vi "20210709_Scan with scanning mirror_draw graph_subVI.vi"(0 "X center (V)":dbl min=-200.0 max=300.0, 1 "Y center (V)":dbl min=-200.0 max=300.0, 2 "Bool Refnum":refnum<vi>, 4 "X Scan range (V)":dbl=0.2 min=-200.0 max=300.0, 5 "Y Scan range (V)":dbl=0.2 min=-200.0 max=300.0, 6 "X data number(Ao1)":i32=150, 7 "Y data number(Ao0)":i32=150, 8 "DigNum Refnum 7":refnum<vi>, 9 "DigNum Refnum 4":refnum<vi>, 10 "DigNum Refnum 3":refnum<vi>, 11 "DigNum Refnum 8":refnum<vi>, 12 "DigNum Refnum 5":refnum<vi>, 13 "DigNum Refnum 6":refnum<vi>, 14 "IntGraph Refnum":refnum<vi>, 18 "DigNum Refnum":refnum<vi>, 19 "DigNum Refnum 2":refnum<vi>) -> (15 "Intensity Graph":dbl[][](graph))   [LabVIEW 2015]
uses:
  Libraries/SR400/Public/Typedefs/Counter.ctl
  <vilib>/Analysis/1siggen.llb/Ramp Pattern by Samples.vi
  <vilib>/Analysis/NI_AALBase.lvlib
  Libraries/SR400/SR400.lvlib
panel:
  in  "file path":path
  out "STOP SCAN":bool
  in  "Count Time Set":dbl[unit]=0.01
  in  "# of average":i32=1
  in  "Dwell time (ms)":i32=2
  in  "Time delay bet. movement\n& measurement (ms)":i32=1
  out "Max Value":dbl format="%#.2p"
  out "Max Y (V)":dbl format="%#.5f"
  out "Max X (V)":dbl format="%#.5f"
  out "Counts":dbl
  out "ao1_V":dbl
  out "ao1_index":i32
  out "ao0_V":dbl
  out "ao0_index":i32
  in  "VISA resource name":refnum<visa-resource-name>="GPIB0::18::INSTR"
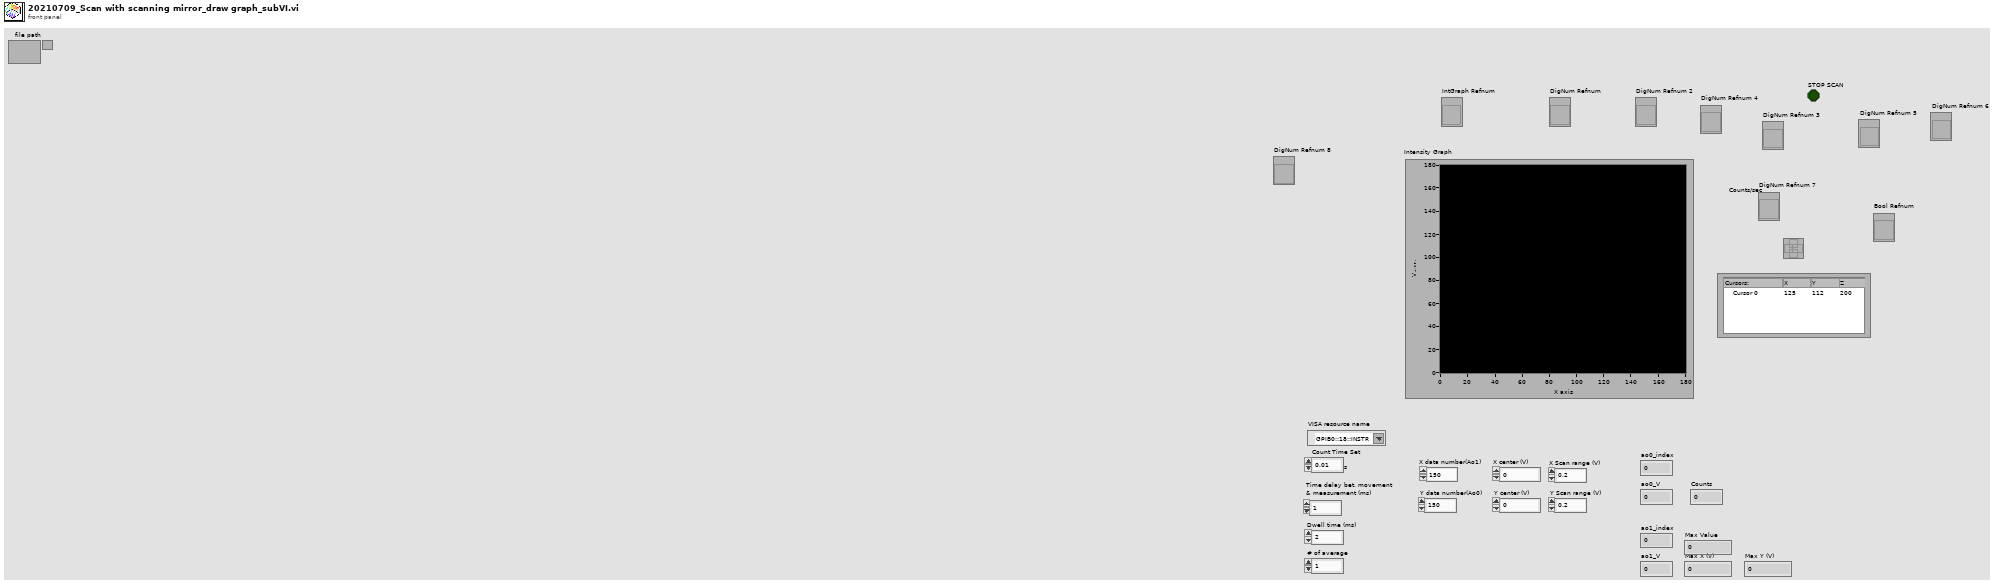
[diagram p1: front panel]
types:
  T1 = enum16{"open", "open or create", "create or replace", "create", "open (read only)"}
  T2 = typedef "SR400.lvlib/Counter.ctl" = enum16{"Counter A", "Counter B", "Counter T"}
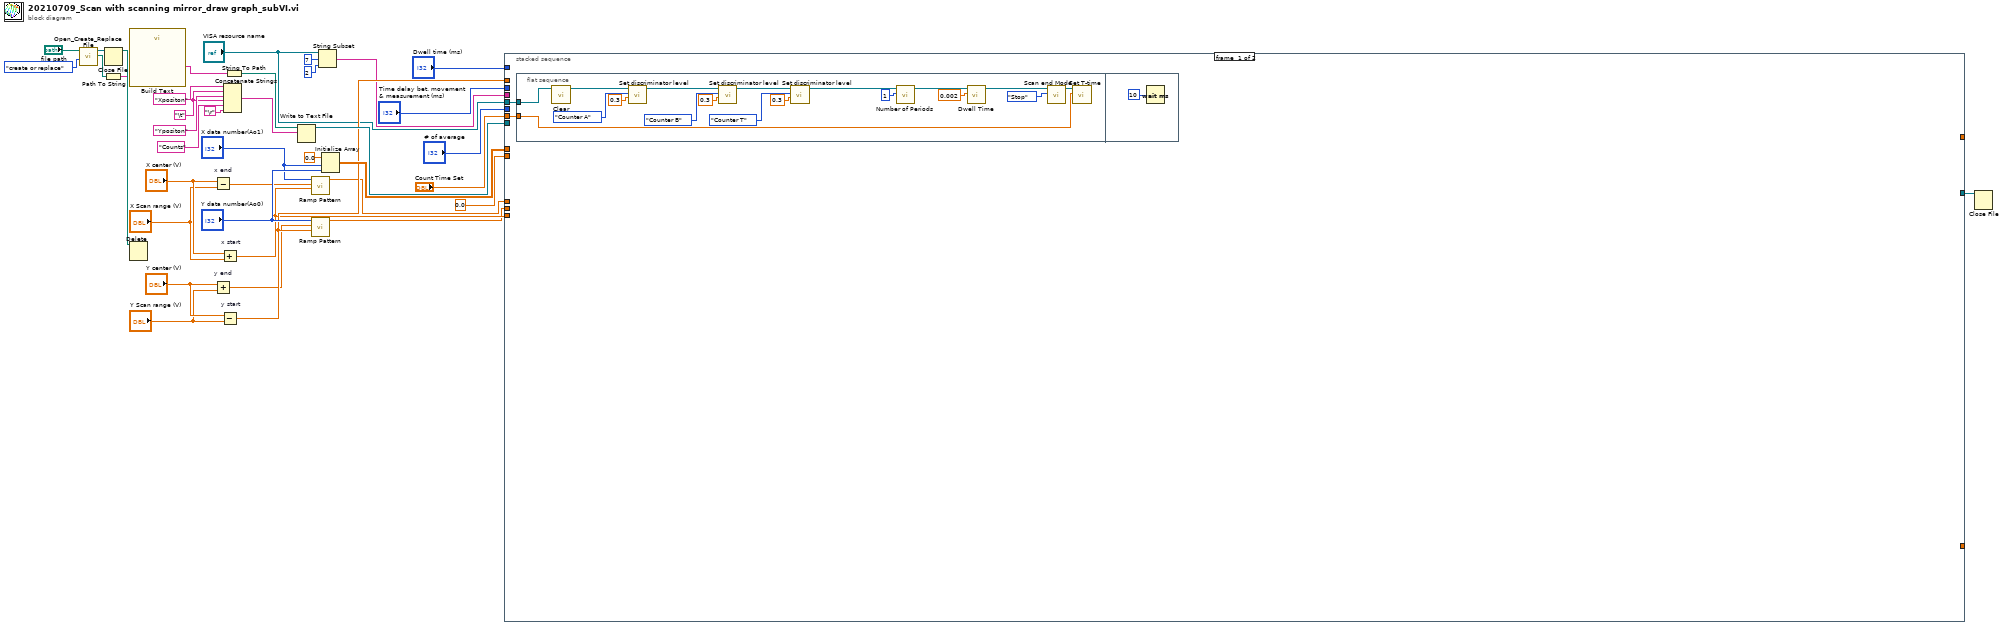
[diagram p0: block diagram]
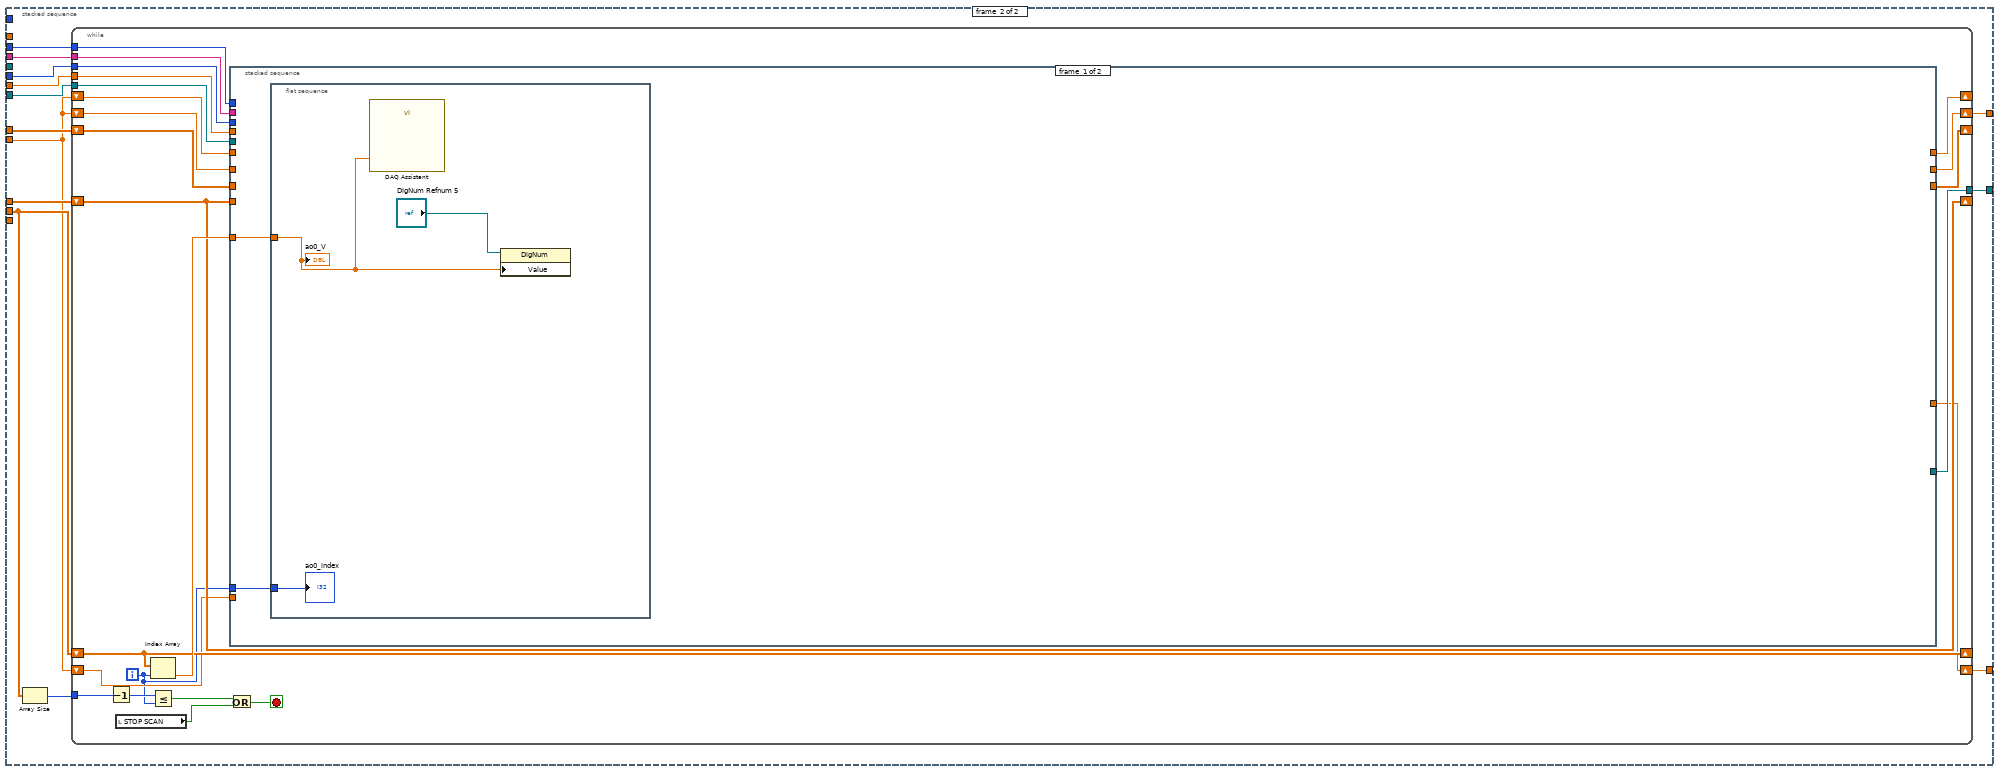
[diagram p2: hidden frame]
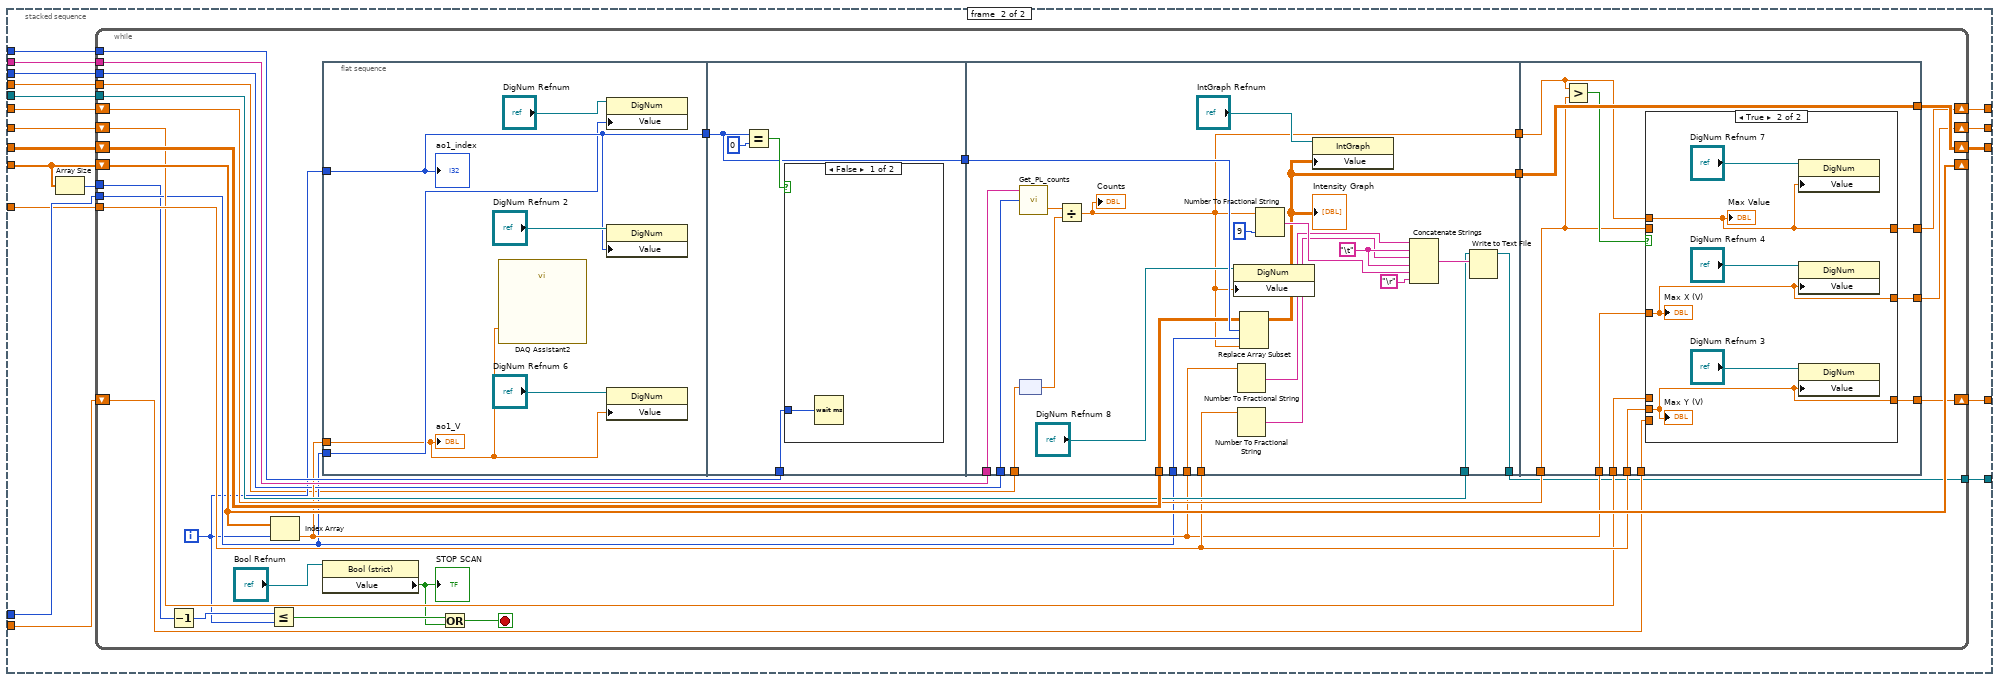
[diagram p3: hidden frame]
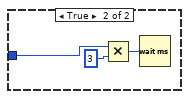
[diagram p4: hidden frame]
diagram:
  w31 = "\t"
  n1 = call <vilib>:"Open_Create_Replace File.vi"("function (open:0)"=T1."create or replace", "file path"="file path") -> ("new file path"=w4:path, "refnum"=w6:refnum<file>)  [unwired: 6 in, 2 out]
  n2 = Path To String(path=w4) -> (string=w3:string)
  n3 = Close File(refnum=w6) -> (path=w5:path)  [unwired: 1 in, 1 out]
  n4 = call "Build Text"("a"=w3) -> ("Result"=w2:string)  [unwired: 13 in, 1 out]
  n5 = Delete(path (use dialog)=w5) -> ()  [unwired: 4 in, 3 out]
  n6 = Subtract "x end"(x="X center (V)", y="X Scan range (V)") -> (x-y=w21:dbl)
  n7 = Add "y end"(x="Y center (V)", y="Y Scan range (V)") -> (x+y=w22:dbl)
  n8 = Add "x start"(x="X center (V)", y="X Scan range (V)") -> (x+y=w20:dbl)
  n9 = Subtract "y start"(x="Y center (V)", y="Y Scan range (V)") -> (x-y=w23:dbl)
  n10 = Concatenate Strings("Xpositon" ("string"), w31, "Ypositon" ("string"), w31, "Counts" ("string"), "\r") -> (w34:string)
  n11 = String To Path(string=w2) -> (path=w1:path)
  n12 = Write to Text File(file (use dialog)=w1, text=w34) -> (refnum out=w28:refnum<file>)  [unwired: 2 in, 2 out]
  n13 = call-poly <vilib>:"Ramp Pattern.vi"("start"=w20, "end"=w21, "samples"="X data number(Ao1)") -> ("Ramp Pattern"=w14:dbl[])  [unwired: 7 in, 1 out]
  n14 = call-poly <vilib>:"Ramp Pattern.vi"("start"=w23, "end"=w22, "samples"="Y data number(Ao0)") -> ("Ramp Pattern"=w13:dbl[])  [unwired: 7 in, 1 out]
  n15 = String Subset(string="VISA resource name", offset (0)=7, length (rest)=2 ("length (rest)")) -> (substring=w10:string)
  n16 = Initialize Array(0.0, "X data number(Ao1)", "Y data number(Ao0)") -> (w35:dbl[][])
  n17 = stacked-sequence {
    tunnel: w13 -> [_ w73]
    tunnel: w14 -> [_ w72]
    tunnel: "Time delay bet. movement\n& measurement (ms)" -> [_ w71]
    tunnel: w10 -> [_ w70]
    tunnel: w35 -> [_ w69]
    tunnel: w28 -> [_ w68]
    tunnel: [_ w67] -> w27
    tunnel: w20 -> [_ _]
    tunnel: w23 -> [_ _]
    tunnel: 0.0 -> [_ w66]
    tunnel: "Dwell time (ms)" -> [_ _]
    tunnel: [_ w65] -> _
    tunnel: [_ w64] -> _
    tunnel: "# of average" -> [_ w63]
    tunnel: "Count Time Set" -> [w41 w61]
    tunnel: "VISA resource name" -> [w40 _]
    frame #0 {
      n18 = flat-sequence {
        tunnel: w41 -> [w43]
        tunnel: w40 -> [w42]
        frame #0 {
          n19 = call "Clear.vi"("VISA resource name"=w42) -> ("VISA resource name out"=w59:refnum<visa-resource-name>)  [unwired: 9 in, 1 out]
          n20 = call "Set discriminator level.vi"("Level (-0.034 V)"=0.3, "Discriminator (def: A)"=Counter."Counter A", "VISA resource name"=w59) -> ("VISA resource name out"=w56:refnum<visa-resource-name>)  [unwired: 7 in, 1 out]
          n21 = call "Set discriminator level.vi"("Level (-0.034 V)"=0.3, "Discriminator (def: A)"=Counter."Counter B", "VISA resource name"=w56) -> ("VISA resource name out"=w53:refnum<visa-resource-name>)  [unwired: 7 in, 1 out]
          n22 = call "Set discriminator level.vi"("Level (-0.034 V)"=0.3, "Discriminator (def: A)"=Counter."Counter T", "VISA resource name"=w53) -> ("VISA resource name out"=w50:refnum<visa-resource-name>)  [unwired: 7 in, 1 out]
          n23 = call "Number of Periods.vi"("# of periods (def: 1)"=1, "VISA resource name"=w50) -> ("VISA resource name out"=w48:refnum<visa-resource-name>)  [unwired: 8 in, 1 out]
          n24 = call "Dwell Time.vi"("Dwell time (0.002 s)"=0.002, "VISA resource name"=w48) -> ("VISA resource name out"=w46:refnum<visa-resource-name>)  [unwired: 8 in, 1 out]
          n25 = call "Scan end Mode.vi"("Scan End Mode (Def: Stop)"=enum16{"Stop", "Start"}."Stop", "VISA resource name"=w46) -> ("VISA resource name out"=w44:refnum<visa-resource-name>)  [unwired: 8 in, 1 out]
          n26 = call "Set T-time.vi"("Count Time Set"=w43, "VISA resource name"=w44) -> ()  [unwired: 5 in, 3 out]
        }
        frame #1 {
          n27 = Wait (ms)(milliseconds to wait=u32 10) -> ()  [unwired: 1 out]
        }
      }
    }
    frame #1 {
      n28 = Array Size(array=w73) -> (size(s)=w62:i32)
      n29 = while {
        shift-right: [w95] -> _
        shift-left: w73 -> [w95]
        shift-right: [w94] -> _
        shift-left: w72 -> [w94]
        tunnel: w71 -> [w93]
        tunnel: w70 -> [w92]
        shift-right: [w89] -> _
        shift-left: w69 -> [w91]
        tunnel: w68 -> [w90]
        tunnel: [w88] -> w67
        shift-right: [w87] -> w64
        shift-left: w66 -> [w82]
        shift-right: [w85] -> _
        shift-left: w66 -> [w83]
        shift-right: [w86] -> w65
        shift-left: w66 -> [w84]
        tunnel: w63 -> [w81]
        tunnel: w62 -> [w80]
        tunnel: w61 -> [w74]
        i -> [w78]
        stop <- w75 stop-if-true
        n30 = Decrement(x=w80) -> (x-1=w79:i32)
        n31 = local read "STOP SCAN"() -> (w76:bool)
        n32 = Index Array(array=w95, index=w78) -> (element=w96:dbl)
        n33 = Less Or Equal?(x=w79, y=w78) -> (x <= y?=w77:bool)
        n34 = stacked-sequence {
          tunnel: w96 -> [w98 w114]
          tunnel: w94 -> [_ w119]
          tunnel: w93 -> [_ w118]
          tunnel: w78 -> [w97 w116]
          tunnel: w92 -> [_ w117]
          tunnel: w91 -> [_ w115]
          tunnel: w90 -> [_ w113]
          tunnel: [_ w112] -> w89
          tunnel: [_ w111] -> w88
          tunnel: [_ w110] -> w87
          tunnel: [_ w109] -> w86
          tunnel: [_ w108] -> w85
          tunnel: w84 -> [_ w107]
          tunnel: w83 -> [_ w106]
          tunnel: w82 -> [_ w105]
          tunnel: w81 -> [_ w104]
          tunnel: w74 -> [_ w102]
          frame #0 {
            n35 = flat-sequence {
              tunnel: w98 -> [w99]
              tunnel: w97 -> [w101]
              frame #0 {
                n36 = call "DAQ Assistant"("data"=w99) -> ()  [unwired: 17 in, 2 out]
                n37 = property class="DigNum"(reference="DigNum Refnum 5", "Value"=w99) -> ()  [unwired: 1 in, 2 out]
                "ao0_V" <- w99
                "ao0_index" <- w101
              }
            }
          }
          frame #1 {
            n38 = Array Size(array=w119) -> (size(s)=w103:i32)
            n39 = while {
              shift-right: [w148] -> _
              shift-left: w119 -> [w148]
              tunnel: w118 -> [w147]
              tunnel: w117 -> [w146]
              tunnel: w116 -> [w128]
              shift-right: [w143] -> w112
              shift-left: w115 -> [w144]
              tunnel: w114 -> [w137]
              tunnel: w113 -> [w142]
              shift-right: [w139] -> w108
              shift-left: w106 -> [w138]
              shift-right: [w135] -> w110
              shift-left: w105 -> [w133]
              shift-right: [w134] -> w109
              shift-left: w107 -> [w132]
              tunnel: [w131] -> w111
              tunnel: w104 -> [w129]
              tunnel: w103 -> [w127]
              tunnel: w102 -> [w120]
              i -> [w125]
              stop <- w123 stop-if-true
              n40 = Decrement(x=w127) -> (x-1=w126:i32)
              n41 = Less Or Equal?(x=w126, y=w125) -> (x <= y?=w124:bool)
              n42 = Index Array(array=w148, index=w125) -> (element=w136:dbl)
              n43 = flat-sequence {
                tunnel: w136 -> [w149]
                tunnel: w125 -> [w152]
                tunnel: [w152] -> w130
                tunnel: w128 -> [w151]
                tunnel: w147 -> [w155]
                tunnel: [w157] -> w145
                tunnel: w130 -> [w157]
                tunnel: w146 -> [w171]
                tunnel: w145 -> [w185]
                tunnel: w128 -> [w184]
                tunnel: w144 -> [w183]
                tunnel: w136 -> [w176]
                tunnel: w137 -> [w175]
                tunnel: w142 -> [w173]
                tunnel: [w168] -> w141
                tunnel: [w164] -> w140
                tunnel: [w172] -> w131
                tunnel: w129 -> [w170]
                tunnel: w120 -> [w165]
                tunnel: [w196] -> w143
                tunnel: w141 -> [w196]
                tunnel: w140 -> [w186]
                tunnel: [w194] -> w139
                tunnel: w138 -> [w187]
                tunnel: w137 -> [w193]
                tunnel: w136 -> [w192]
                tunnel: [w191] -> w135
                tunnel: [w190] -> w134
                tunnel: w133 -> [w189]
                tunnel: w132 -> [w188]
                frame #0 {
                  n44 = call "DAQ Assistant2"("data"=w149) -> ()  [unwired: 17 in, 2 out]
                  n45 = property class="DigNum"(reference="DigNum Refnum", "Value"=w151) -> ()  [unwired: 1 in, 2 out]
                  n46 = property class="DigNum"(reference="DigNum Refnum 2", "Value"=w152) -> ()  [unwired: 1 in, 2 out]
                  n47 = property class="DigNum"(reference="DigNum Refnum 6", "Value"=w149) -> ()  [unwired: 1 in, 2 out]
                  "ao1_V" <- w149
                  "ao1_index" <- w152
                }
                frame #1 {
                  n48 = Equal?(x=w157, y=0) -> (x = y?=w158:bool)
                  n49 = case shown="False" w158 {
                    tunnel: w155 -> [w159 w161]
                    frame False {
                      n50 = Wait (ms)(milliseconds to wait=w159) -> ()  [unwired: 1 out]
                    }
                    frame True {
                      n51 = Multiply(x=w161, y=3) -> (x*y=w162:i32)
                      n52 = Wait (ms)(milliseconds to wait=w162) -> ()  [unwired: 1 out]
                    }
                  }
                }
                frame #2 {
                  w182 = "\t"
                  n53 = call "Get_PL_counts.vi"("# of average"=w170, "SR400 GPIB Address"=w171) -> ("Averaged counts"=w163:dbl)  [unwired: 2 in]
                  n54 = node(w165) -> (w166:dbl)
                  n55 = Divide(x=w163, y=w166) -> (x/y=w164:dbl)
                  "Counts" <- w164
                  n56 = property class="DigNum"(reference="DigNum Refnum 8", "Value"=w164) -> ()  [unwired: 1 in, 2 out]
                  n57 = Number To Fractional String(number=w176) -> (F-format string=w177:string)  [unwired: 3 in]
                  n58 = Number To Fractional String(number=w175) -> (F-format string=w174:string)  [unwired: 3 in]
                  n59 = Replace Array Subset(array=w183, new element=w164, index (row)=w185, index (col)=w184) -> (w168:dbl[][])
                  "Intensity Graph" <- w168
                  n60 = Number To Fractional String(number=w164, precision (6)=i16 9) -> (F-format string=w178:string)  [unwired: 2 in]
                  n61 = property class="IntGraph"(reference="IntGraph Refnum", "Value"=w168) -> ()  [unwired: 1 in, 2 out]
                  n62 = Concatenate Strings(w177, w182, w174, w182, w178, "\r") -> (w180:string)
                  n63 = Write to Text File(file (use dialog)=w173, text=w180) -> (refnum out=w172:refnum<file>)  [unwired: 2 in, 2 out]
                }
                frame #3 {
                  n64 = Greater?(x=w186, y=w187) -> (0:w195:bool)
                  n65 = case shown="True" w195 {
                    tunnel: w186 -> [_ w200]
                    tunnel: [w199 w200] -> w194
                    tunnel: w187 -> [w199 _]
                    tunnel: w193 -> [_ w202]
                    tunnel: w192 -> [_ w204]
                    tunnel: [w198 w202] -> w191
                    tunnel: [w197 w204] -> w190
                    tunnel: w189 -> [w198 _]
                    tunnel: w188 -> [w197 _]
                    frame False {
                    }
                    frame True {
                      n66 = property class="DigNum"(reference="DigNum Refnum 7", "Value"=w200) -> ()  [unwired: 1 in, 2 out]
                      n67 = property class="DigNum"(reference="DigNum Refnum 4", "Value"=w204) -> ()  [unwired: 1 in, 2 out]
                      n68 = property class="DigNum"(reference="DigNum Refnum 3", "Value"=w202) -> ()  [unwired: 1 in, 2 out]
                      "Max Value" <- w200
                      "Max Y (V)" <- w202
                      "Max X (V)" <- w204
                    }
                  }
                }
              }
              n69 = property class="Bool (strict)"(reference="Bool Refnum") -> ("Value"=w121:bool)  [unwired: 1 in, 2 out]
              "STOP SCAN" <- w121
              n70 = Or(x=w124, y=w121) -> (x .or. y?=w123:bool)
            }
          }
        }
        n71 = Or(x=w77, y=w76) -> (x .or. y?=w75:bool)
      }
    }
  }
  n72 = Close File(refnum=w27) -> ()  [unwired: 1 in, 2 out]
